vi "Convert XML to Option Cluster.vi"(8 "CORE Options 2":T2, 11 "Feature":T1(array[cluster])=[{"#attributes"={"Name"="CORE", "Value"="T"}}, {"#attributes"={"Name"="EMITTER", "Value"="T"}}, {"#attributes"={"Name"="INTERFERENCE", "Value"="T"}}, {"#attributes"={"Name"="FCC", "Value"="T"}}, {"#attributes"={"Name"="SCHEDULER", "Value"="T"}}, {"#attributes"={"Name"="DRIVE", "Value"=""}}, {"#attributes"={"Name"="US", "Value"="T"}}, {"#attributes"={"Name"="EUROPE", "Value"=""}}, {"#attributes"={"Name"="CHINA", "Value"=""}}, {"#attributes"={"Name"="AFRICA", "Value"=""}}, {"#attributes"={"Name"="NORTH-SOUTH", "Value"=""}}, {"#attributes"={"Name"="10", "Value"=""}}, {"#attributes"={"Name"="25", "Value"=""}}, {"#attributes"={"Name"="50", "Value"=""}}, {"#attributes"={"Name"="ADVANTEST", "Value"=""}}, {"#attributes"={"Name"="AGILENT", "Value"=""}}, {"#attributes"={"Name"="ANRITSU", "Value"=""}}, {"#attributes"={"Name"="ROHDE", "Value"=""}}, {"#attributes"={"Name"="WILLTEK", "Value"=""}}, {"#attributes"={"Name"="NETTEK", "Value"=""}}, {"#attributes"={"Name"="ICOM", "Value"=""}}]) -> (0 "Feature 2":T1(array[cluster])=[{"#attributes"={"Name"="CORE", "Value"="T"}}, {"#attributes"={"Name"="EMITTER", "Value"="T"}}, {"#attributes"={"Name"="INTERFERENCE", "Value"="T"}}, {"#attributes"={"Name"="FCC", "Value"="T"}}, {"#attributes"={"Name"="SCHEDULER", "Value"="T"}}, {"#attributes"={"Name"="DRIVE", "Value"=""}}, {"#attributes"={"Name"="US", "Value"="T"}}, {"#attributes"={"Name"="EUROPE", "Value"=""}}, {"#attributes"={"Name"="CHINA", "Value"=""}}, {"#attributes"={"Name"="AFRICA", "Value"=""}}, {"#attributes"={"Name"="NORTH-SOUTH", "Value"=""}}, {"#attributes"={"Name"="10", "Value"=""}}, {"#attributes"={"Name"="25", "Value"=""}}, {"#attributes"={"Name"="50", "Value"=""}}, {"#attributes"={"Name"="ADVANTEST", "Value"=""}}, {"#attributes"={"Name"="AGILENT", "Value"=""}}, {"#attributes"={"Name"="ANRITSU", "Value"=""}}, {"#attributes"={"Name"="ROHDE", "Value"=""}}, {"#attributes"={"Name"="WILLTEK", "Value"=""}}, {"#attributes"={"Name"="NETTEK", "Value"=""}}, {"#attributes"={"Name"="ICOM", "Value"=""}}], 1 "String":string, 3 "CORE Options":T2)   [LabVIEW 2011]
uses:
  CORE Options.ctt
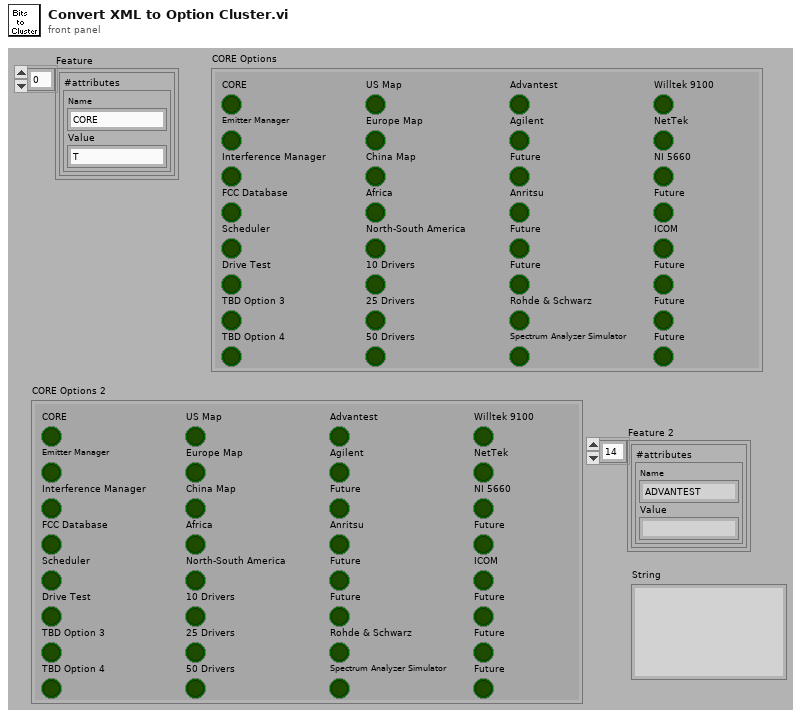
[diagram p1: front panel]
types:
  T1 = cluster{"#attributes":cluster{"Name":string, "Value":string}}[]
  T2 = typedef "CORE Options.ctt" = cluster{"CORE":bool, "Emitter Manager":bool, "Interference Manager":bool, "FCC Database":bool, "Scheduler":bool, "Drive Test":bool, "TBD Option 3":bool, "TBD Option 4":bool, "US Map":bool, "Europe Map":bool, "China Map":bool, "Africa":bool, "North-South America":bool, "10 Drivers":bool, "25 Drivers":bool, "50 Drivers":bool, "Advantest":bool, "Agilent":bool, "Future":bool, "Anritsu":bool, "Future":bool, "Future":bool, "Rohde & Schwarz":bool, "Spectrum Analyzer Simulator":bool, "Willtek 9100":bool, "NetTek":bool, "NI 5660":bool, "Future":bool, "ICOM":bool, "Future":bool, "Future":bool, "Future":bool}
  T3 = cluster{"#attributes":cluster{"Name":string, "Value":string}}
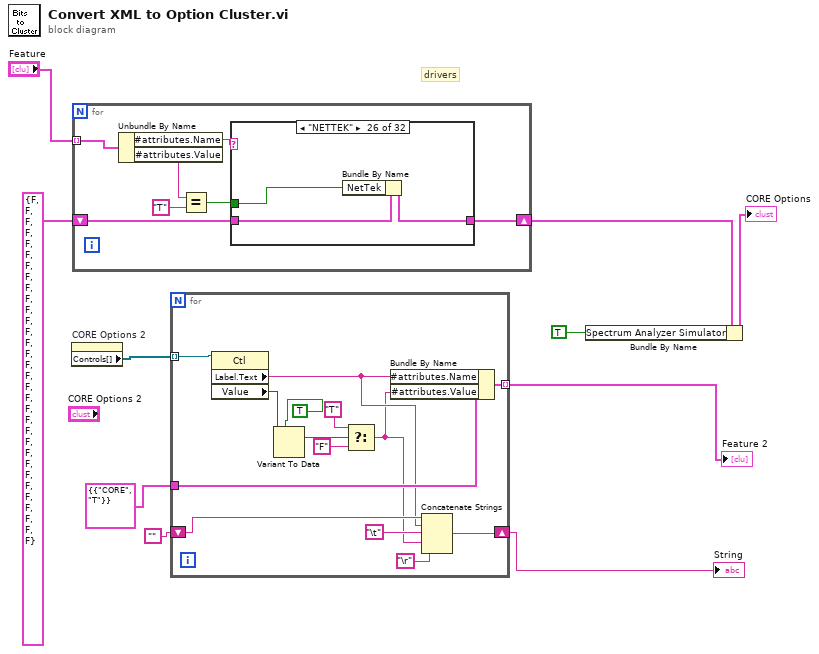
[diagram p0: block diagram]
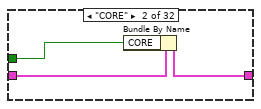
[diagram p3: hidden frame]
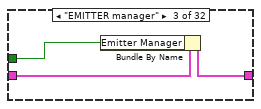
[diagram p4: hidden frame]
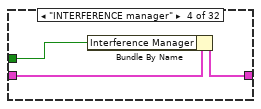
[diagram p5: hidden frame]
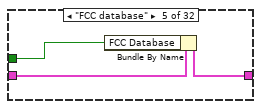
[diagram p6: hidden frame]
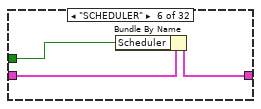
[diagram p7: hidden frame]
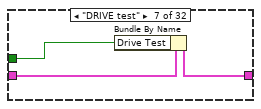
[diagram p8: hidden frame]
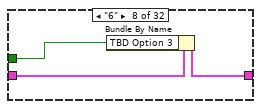
[diagram p9: hidden frame]
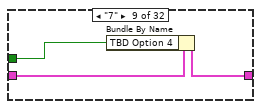
[diagram p10: hidden frame]
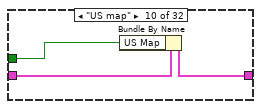
[diagram p11: hidden frame]
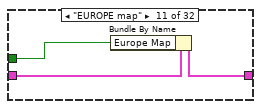
[diagram p12: hidden frame]
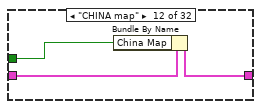
[diagram p13: hidden frame]
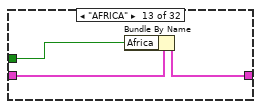
[diagram p14: hidden frame]
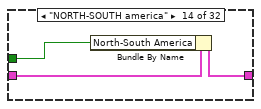
[diagram p15: hidden frame]
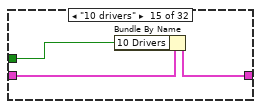
[diagram p16: hidden frame]
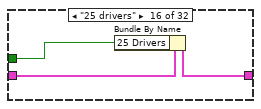
[diagram p17: hidden frame]
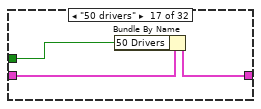
[diagram p18: hidden frame]
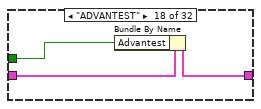
[diagram p19: hidden frame]
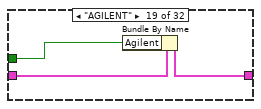
[diagram p20: hidden frame]
diagram:
  # "drivers"
  n1 = property on="CORE Options 2" class="Clust (strict)"() -> ("Controls[]"=w5:refnum<vi>[])  [unwired: 2 in, 2 out]
  n2 = for {
    shift-right: [w16] -> w7
    shift-left: T2 {"CORE"=FALSE, "Emitter Manager"=FALSE, "Interference Manager"=FALSE, "FCC Database"=FALSE, "Scheduler"=FALSE, "Drive Test"=FALSE, "TBD Option 3"=FALSE, "TBD Option 4"=FALSE, "US Map"=FALSE, "Europe Map"=FALSE, "China Map"=FALSE, "Africa"=FALSE, "North-South America"=FALSE, "10 Drivers"=FALSE, "25 Drivers"=FALSE, "50 Drivers"=FALSE, "Advantest"=FALSE, "Agilent"=FALSE, "Future"=FALSE, "Anritsu"=FALSE, "Future"=FALSE, "Future"=FALSE, "Rohde & Schwarz"=FALSE, "Spectrum Analyzer Simulator"=FALSE, "Willtek 9100"=FALSE, "NetTek"=FALSE, "NI 5660"=FALSE, "Future"=FALSE, "ICOM"=FALSE, "Future"=FALSE, "Future"=FALSE, "Future"=FALSE} ("CORE Options") -> [w17]
    tunnel: "Feature" -> [w15] mode=indexing
    n3 = Unbundle By Name(w15) -> ("#attributes.Name"=w14:string, "#attributes.Value"=w12:string)
    n4 = Equal?(x=w12, y="T") -> (x = y?=w13:bool)
    n5 = case shown="\"NETTEK\"" w14 {
      tunnel: w13 -> [_ w19 w22 w25 w28 w31 w34 w37 w40 w43 w46 w49 w52 w55 w58 w61 w64 w67 w70 w73 w76 w79 w82 w85 w88 w91 w94 w97 w100 w103 w106 w109]
      tunnel: w17 -> [w18 w21 w24 w27 w30 w33 w36 w39 w42 w45 w48 w51 w54 w57 w60 w63 w66 w69 w72 w75 w78 w81 w84 w87 w90 w93 w96 w99 w102 w105 w108 w111]
      tunnel: [w18 w20 w23 w26 w29 w32 w35 w38 w41 w44 w47 w50 w53 w56 w59 w62 w65 w68 w71 w74 w77 w80 w83 w86 w89 w92 w95 w98 w101 w104 w107 w110] -> w16
      frame Default {
      }
      frame "CORE" {
        n6 = Bundle By Name(cluster=w21, "CORE"=w19) -> (w20:T2)
      }
      frame "EMITTER manager" {
        n7 = Bundle By Name(cluster=w24, "Emitter Manager"=w22) -> (w23:T2)
      }
      frame "INTERFERENCE manager" {
        n8 = Bundle By Name(cluster=w27, "Interference Manager"=w25) -> (w26:T2)
      }
      frame "FCC database" {
        n9 = Bundle By Name(cluster=w30, "FCC Database"=w28) -> (w29:T2)
      }
      frame "SCHEDULER" {
        n10 = Bundle By Name(cluster=w33, "Scheduler"=w31) -> (w32:T2)
      }
      frame "DRIVE test" {
        n11 = Bundle By Name(cluster=w36, "Drive Test"=w34) -> (w35:T2)
      }
      frame "6" {
        n12 = Bundle By Name(cluster=w39, "TBD Option 3"=w37) -> (w38:T2)
      }
      frame "7" {
        n13 = Bundle By Name(cluster=w42, "TBD Option 4"=w40) -> (w41:T2)
      }
      frame "US map" {
        n14 = Bundle By Name(cluster=w45, "US Map"=w43) -> (w44:T2)
      }
      frame "EUROPE map" {
        n15 = Bundle By Name(cluster=w48, "Europe Map"=w46) -> (w47:T2)
      }
      frame "CHINA map" {
        n16 = Bundle By Name(cluster=w51, "China Map"=w49) -> (w50:T2)
      }
      frame "AFRICA" {
        n17 = Bundle By Name(cluster=w54, "Africa"=w52) -> (w53:T2)
      }
      frame "NORTH-SOUTH america" {
        n18 = Bundle By Name(cluster=w57, "North-South America"=w55) -> (w56:T2)
      }
      frame "10 drivers" {
        n19 = Bundle By Name(cluster=w60, "10 Drivers"=w58) -> (w59:T2)
      }
      frame "25 drivers" {
        n20 = Bundle By Name(cluster=w63, "25 Drivers"=w61) -> (w62:T2)
      }
      frame "50 drivers" {
        n21 = Bundle By Name(cluster=w66, "50 Drivers"=w64) -> (w65:T2)
      }
      frame "ADVANTEST" {
        n22 = Bundle By Name(cluster=w69, "Advantest"=w67) -> (w68:T2)
      }
      frame "AGILENT" {
        n23 = Bundle By Name(cluster=w72, "Agilent"=w70) -> (w71:T2)
      }
      frame "18" {
        n24 = Bundle By Name(cluster=w75, "Future"=w73) -> (w74:T2)
      }
      frame "ANRITSU" {
        n25 = Bundle By Name(cluster=w78, "Anritsu"=w76) -> (w77:T2)
      }
      frame "20" {
        n26 = Bundle By Name(cluster=w81, "Future"=w79) -> (w80:T2)
      }
      frame "21" {
        n27 = Bundle By Name(cluster=w84, "Future"=w82) -> (w83:T2)
      }
      frame "Rohde & Schwarz" {
        n28 = Bundle By Name(cluster=w87, "Rohde & Schwarz"=w85) -> (w86:T2)
      }
      frame "WILLTEK 9100" {
        n29 = Bundle By Name(cluster=w90, "Willtek 9100"=w88) -> (w89:T2)
      }
      frame "NETTEK" {
        n30 = Bundle By Name(cluster=w93, "NetTek"=w91) -> (w92:T2)
      }
      frame "26" {
        n31 = Bundle By Name(cluster=w96, "NI 5660"=w94) -> (w95:T2)
      }
      frame "27" {
        n32 = Bundle By Name(cluster=w99, "Future"=w97) -> (w98:T2)
      }
      frame "ICOM" {
        n33 = Bundle By Name(cluster=w102, "ICOM"=w100) -> (w101:T2)
      }
      frame "29" {
        n34 = Bundle By Name(cluster=w105, "Future"=w103) -> (w104:T2)
      }
      frame "30" {
        n35 = Bundle By Name(cluster=w108, "Future"=w106) -> (w107:T2)
      }
      frame "31" {
        n36 = Bundle By Name(cluster=w111, "Future"=w109) -> (w110:T2)
      }
    }
  }
  n37 = for {
    tunnel: w5 -> [w125] mode=indexing
    tunnel: T3 {"#attributes"={"Name"="CORE", "Value"="T"}} -> [w124]
    tunnel: [w123] -> w3 mode=indexing
    shift-right: [w112] -> w1
    shift-left: "" -> [w115]
    n38 = property class="Ctl"(reference=w125) -> ("Label.Text"=w114:string, "Value"=w122:variant)  [unwired: 1 in, 2 out]
    n39 = Variant To Data(type=TRUE, Variant=w122) -> (data=w120:bool)  [unwired: 1 in, 1 out]
    n40 = Select(t="T" ("y"), s=w120, f="F") -> (s? t:f=w113:string)
    n41 = Bundle By Name(cluster=w124, "#attributes.Name"=w114, "#attributes.Value"=w113) -> (w123:T3)
    n42 = Concatenate Strings(w115, w114, "\t", w113, "\r") -> (w112:string)
  }
  "Feature 2" <- w3
  "String" <- w1
  n43 = Bundle By Name(cluster=w7, "Spectrum Analyzer Simulator"=TRUE) -> (→"CORE Options":T2)
